vi "StitchingModeOffset_KJM.vi"(9 "Data In":dbl[][][](array[numeric])) -> (2 "Stitched Data Out":dbl[][](array[numeric]))   [LabVIEW 2020]
doc: "Stitches spectra based on simple cut-off modus."
uses:
  4c98e68f-fed8-44bd-a6f6-c5aabdf5d44d.vi
  <vilib>/numeric/Random Number (Range) U64.vi
panel:
  out "y2? overlap":dbl[][](array[numeric])
  out "y2 ? overlap":dbl[][](array[numeric])
  out "y1 ? overlap":dbl[][](array[numeric])
  out "y1 ? overlap":dbl[][](array[numeric])
  out "x2 after overlap":dbl[](array[numeric])
  out "x2 before overlap":dbl[](array[numeric])
  out "x1 after overlap":dbl[](array[numeric])
  out "x1 before overlap":dbl[](array[numeric])
  out "y2 after overlap 2":dbl[][](array[numeric])
  out "y1 after overlap":dbl[][](array[numeric])
  out "x1":dbl[](array[numeric])
  out "x2":dbl[](array[numeric])
  out "appended array 4":dbl[][](array[numeric])
  out "appended array 3":dbl[][](array[numeric])
  out "appended array 2":u64[][](array[numeric])
  out "appended array":dbl[][][](array[numeric])
  out "y2":dbl[][](array[numeric])
  out "y1":dbl[][](array[numeric])
  out "deleted portion":dbl[][](array[numeric])
  out "array w/ subset deleted":dbl[][](array[numeric])
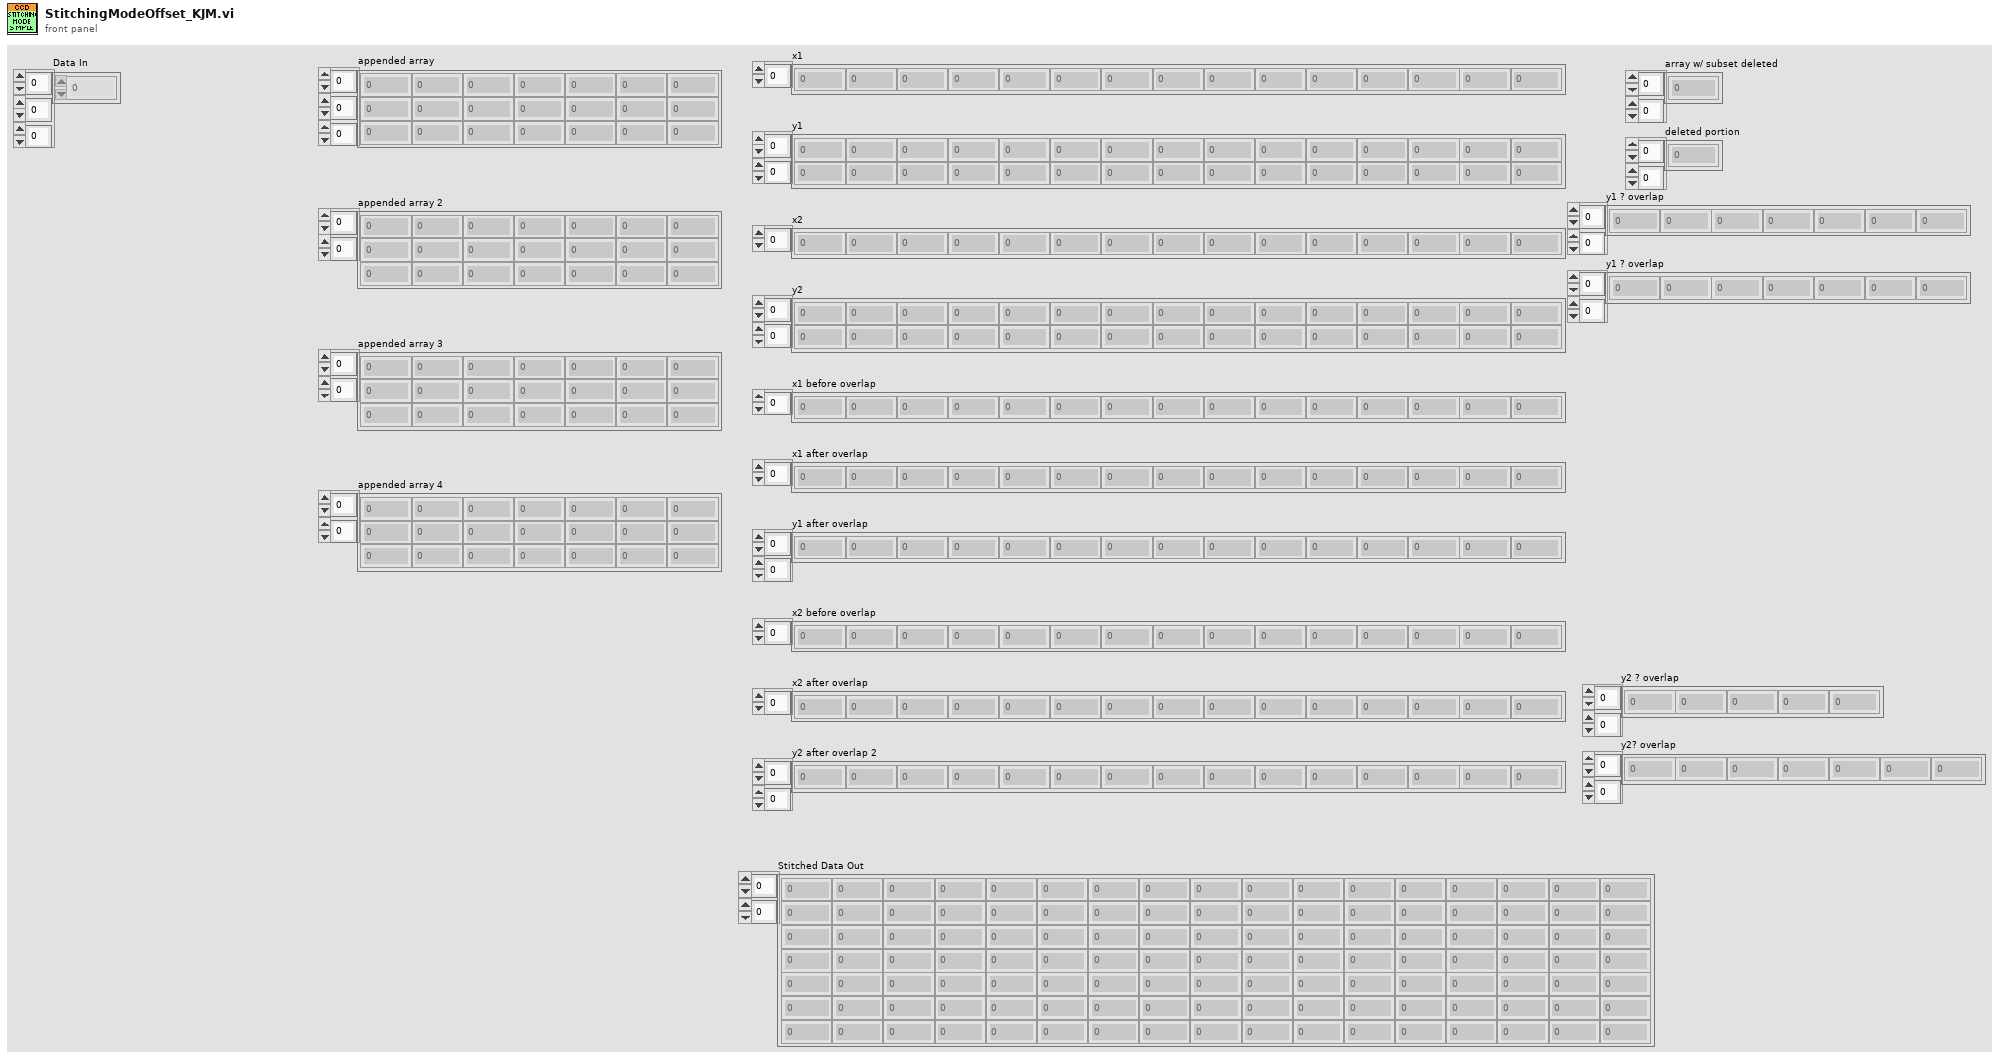
[diagram p1: front panel]
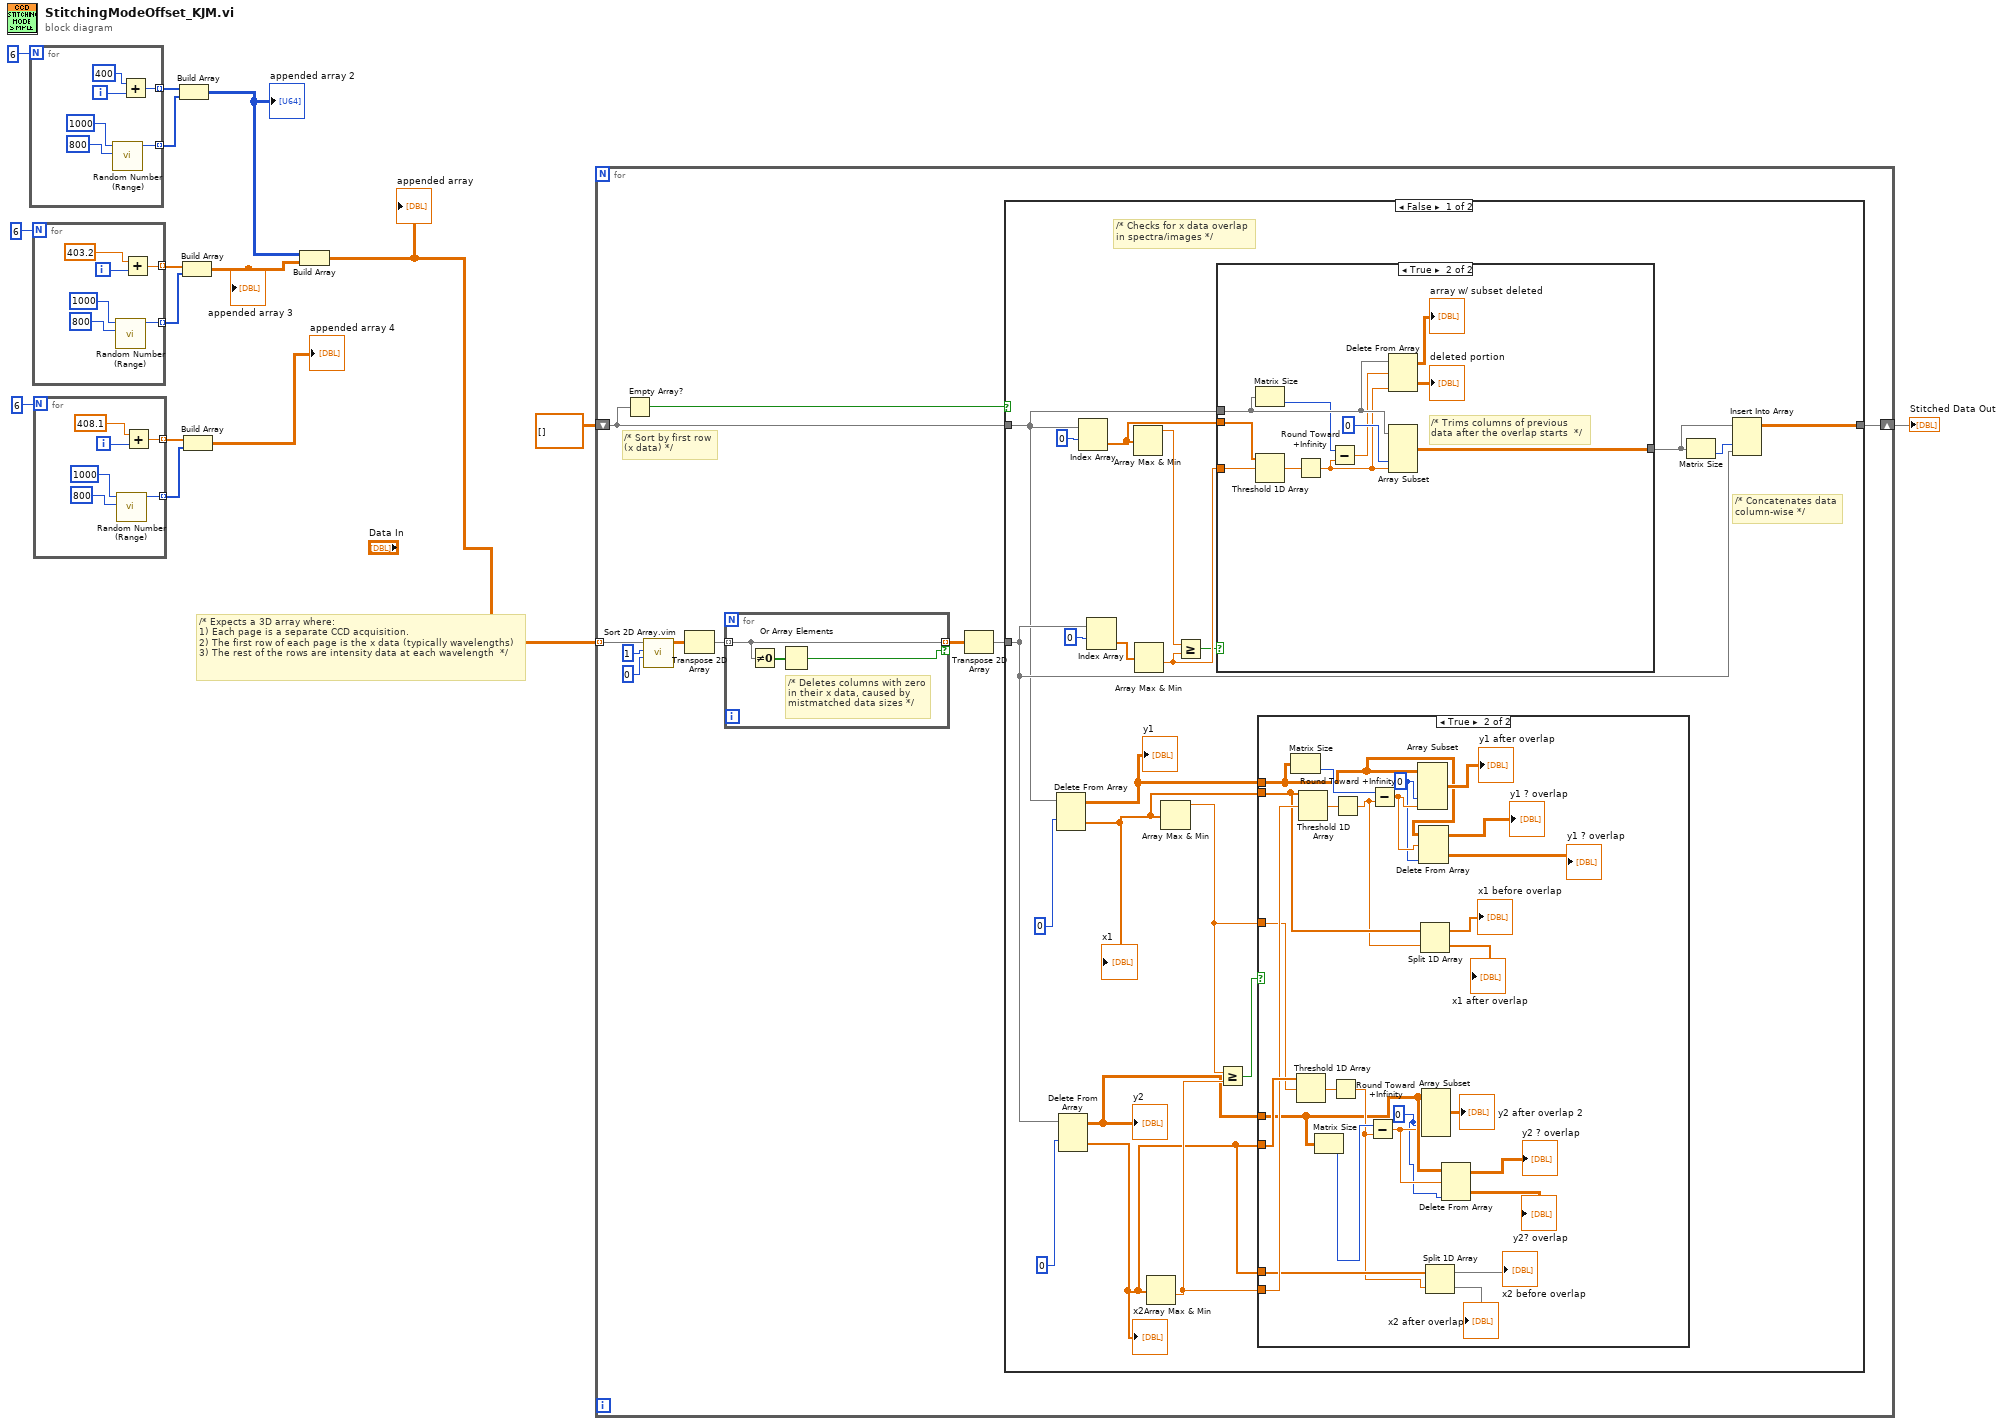
[diagram p0: block diagram]
diagram:
  # "/* Expects a 3D array where:\n1) Each page is a separate CCD acquisition.\n2) The first row of each page is the x data (typically wavelengths)\n3) The rest of the rows are intensity data at each wavelength  */"
  n1 = for {
    N: 6 -> [_]
    tunnel: [w17] -> w12 mode=indexing
    tunnel: [w16] -> w11 mode=indexing
    i -> [w19]
    n2 = call-poly <vilib>:"Random Number (Range).vi"("lower bound (0)"=u64 800, "upper bound (100)"=u64 1000) -> ("number"=w16:u64)  [unwired: 9 in]
    n3 = Add(x=400, y=w19) -> (x+y=w17:i32)
  }
  n4 = for {
    N: 6 -> [_]
    tunnel: [w24] -> w8 mode=indexing
    tunnel: [w23] -> w7 mode=indexing
    i -> [w25]
    n5 = call-poly <vilib>:"Random Number (Range).vi"("lower bound (0)"=u64 800, "upper bound (100)"=u64 1000) -> ("number"=w23:u64)  [unwired: 9 in]
    n6 = Add(x=403.2, y=w25) -> (x+y=w24:dbl)
  }
  n7 = for {
    N: 6 -> [_]
    tunnel: [w30] -> w5 mode=indexing
    tunnel: [w29] -> w4 mode=indexing
    i -> [w31]
    n8 = call-poly <vilib>:"Random Number (Range).vi"("lower bound (0)"=u64 800, "upper bound (100)"=u64 1000) -> ("number"=w29:u64)  [unwired: 9 in]
    n9 = Add(x=408.1, y=w31) -> (x+y=w30:dbl)
  }
  n10 = Build Array(w12, w11) -> (w10:u64[][])
  "appended array 2" <- w10
  n11 = Build Array(w8, w7) -> (w3:dbl[][])
  "appended array 3" <- w3
  n12 = Build Array(w5, w4) -> (→"appended array 4":dbl[][])
  n13 = Build Array(w10, w3) -> (w1:dbl[][][])
  "appended array" <- w1
  n14 = for {
    tunnel: w1 -> [w36] mode=indexing
    shift-right: [w43] -> w15
    shift-left: dbl[][] [] ("Empty Array") -> [w41]
    # "/* Sort by first row \n(x data) */"
    n15 = Empty Array?(array=w41) -> (empty?=w42:bool)
    n16 = call "Sort 2D Array.vim"("index"=0, "dimension to index (column)"=1 ("index"), "2D array"=w36) -> ("sorted 2D array"=w35:dbl[][])  [unwired: 7 in, 1 out]
    n17 = Transpose 2D Array(2D array=w35) -> (transposed array=w40:dbl[][])
    n18 = for {
      tunnel: w40 -> [w45] mode=indexing
      tunnel: [w45] -> w39 mode=indexing if=w46
      # "/* Deletes columns with zero\nin their x data, caused by\nmistmatched data sizes */"
      n19 = Not Equal To 0?(x=w45) -> (x != 0?=w44:bool[])
      n20 = Or Array Elements(Boolean array=w44) -> (logical OR=w46:bool)
    }
    n21 = Transpose 2D Array(2D array=w39) -> (transposed array=w34:dbl[][])
    n22 = case shown="False" w42 {
      tunnel: [w58 w107] -> w43
      tunnel: w34 -> [w57 w107]
      tunnel: w41 -> [w56 _]
      frame False {
        # "/* Concatenates data \ncolumn-wise */"
        # "/* Checks for x data overlap \nin spectra/images */"
        n23 = Delete From Array(array=w56, index (row)=0) -> (deleted portion=w52:dbl[], array with subset deleted=w49:dbl[][])  [unwired: 2 in]
        "y1" <- w49
        "x1" <- w52
        n24 = Delete From Array(array=w57, index (row)=0) -> (deleted portion=w47:dbl[], array with subset deleted=w48:dbl[][])  [unwired: 2 in]
        "y2" <- w48
        "x2" <- w47
        n25 = Index Array(array=w56, index (row)=0) -> (element=w63:dbl[])  [unwired: 1 in]
        n26 = Index Array(array=w57, index (row)=0) -> (element=w65:dbl[])  [unwired: 1 in]
        n27 = Array Max & Min(array=w63) -> (max value=w62:dbl)  [unwired: 3 out]
        n28 = Array Max & Min(array=w65) -> (min value=w61:dbl)  [unwired: 3 out]
        n29 = Array Max & Min(array=w47) -> (min value=w51:dbl)  [unwired: 3 out]
        n30 = Array Max & Min(array=w52) -> (max value=w50:dbl)  [unwired: 3 out]
        n31 = Greater Or Equal?(x=w62, y=w61) -> (x >= y?=w60:bool)
        n32 = case shown="True" w60 {
          tunnel: w56 -> [w95 w101]
          tunnel: [w95 w105] -> w59
          tunnel: w61 -> [_ w104]
          tunnel: w63 -> [_ w103]
          frame False {
            # "/* Passes previous data if \nthere is no overlap */"
          }
          frame True {
            # "/* Trims columns of previous \ndata after the overlap starts  */"
            n33 = Matrix Size(0:w101) -> (2:w100:i32)  [unwired: 1 out]
            n34 = Threshold 1D Array(2:w104, 3:w103) -> (0:w102:dbl)  [unwired: 1 in]
            n35 = Round Toward +Infinity(x=w102) -> (ceil(x): smallest int >= x=w98:dbl)
            n36 = Subtract(x=w100, y=w98) -> (x-y=w99:dbl)
            n37 = Delete From Array(array=w101, length=w99, index (col)=w98) -> (deleted portion=→"deleted portion":dbl[][], array with subset deleted=→"array w/ subset deleted":dbl[][])  [unwired: 1 in]
            n38 = Array Subset(array=w101, index (col)=0 ("index"), length (col)=w98) -> (w105:dbl[][])  [unwired: 2 in]
          }
        }
        n39 = Greater Or Equal?(x=w50, y=w51) -> (x >= y?=w53:bool)
        n40 = case shown="True" w53 {
          tunnel: w52 -> [_ w85]
          tunnel: w47 -> [_ w92]
          tunnel: w51 -> [_ w91]
          tunnel: w50 -> [_ w90]
          tunnel: w49 -> [_ w77]
          tunnel: w48 -> [_ w78]
          tunnel: w47 -> [_ w82]
          frame False {
          }
          frame True {
            w69 = 0 ("index")
            w68 = 0 ("index")
            n41 = Matrix Size(0:w77) -> (2:w89:i32)  [unwired: 1 out]
            n42 = Threshold 1D Array(2:w90, 3:w92) -> (0:w93:dbl)  [unwired: 1 in]
            n43 = Threshold 1D Array(2:w91, 3:w85) -> (0:w94:dbl)  [unwired: 1 in]
            n44 = Matrix Size(0:w78) -> (2:w86:i32)  [unwired: 1 out]
            n45 = Round Toward +Infinity(x=w93) -> (ceil(x): smallest int >= x=w79:dbl)
            n46 = Round Toward +Infinity(x=w94) -> (ceil(x): smallest int >= x=w71:dbl)
            n47 = Subtract(x=w86, y=w79) -> (x-y=w72:dbl)
            n48 = Subtract(x=w89, y=w71) -> (x-y=w70:dbl)
            n49 = Array Subset(array=w77, index (col)=w68, length (col)=w70) -> (→"y1 after overlap":dbl[][])  [unwired: 2 in]
            n50 = Delete From Array(array=w77, length=w70, index (col)=w68) -> (deleted portion=→"y1 ? overlap":dbl[][], array with subset deleted=→"y1 ? overlap":dbl[][])  [unwired: 1 in]
            n51 = Split 1D Array(array=w85, index=w71) -> (first subarray=→"x1 before overlap":dbl[], second subarray=→"x1 after overlap":dbl[])
            n52 = Array Subset(array=w78, index (col)=w69, length (col)=w72) -> (→"y2 after overlap 2":dbl[][])  [unwired: 2 in]
            n53 = Split 1D Array(array=w82, index=w79) -> (first subarray=→"x2 before overlap":dbl[], second subarray=→"x2 after overlap":dbl[])
            n54 = Delete From Array(array=w78, length=w72, index (col)=w69) -> (deleted portion=→"y2? overlap":dbl[][], array with subset deleted=→"y2 ? overlap":dbl[][])  [unwired: 1 in]
          }
        }
        n55 = Matrix Size(0:w59) -> (2:w64:i32)  [unwired: 1 out]
        n56 = Insert Into Array(array=w59, index (col)=w64, new element=w57) -> (w58:dbl[][])  [unwired: 1 in]
      }
      frame True {
        # "/* This case will run on the first loop iteration */"
      }
    }
  }
  "Stitched Data Out" <- w15
